vi "child 3 define test.vi"   [LabVIEW 2020, in "Unit Tests for Runner.lvclass"]
uses:
  Unit Tests for Runner.lvclass
  classes/Test/Test.lvclass
  classes/Assert/Assert.lvclass
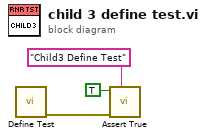
[diagram p0: block diagram]
diagram:
  n1 = call "Define Test.vi"() -> ("error out"=w1:errorcluster)  [unwired: 10 in, 1 out]
  n2 = call "Assert True.vi"("Label"="Child3 Define Test", "error in (no error)"=w1, "True?"=TRUE) -> ()  [unwired: 7 in, 2 out]
